vi "Test Get Report Path.vi"(8 "error in (no error)":errorcluster, 11 "Configuration Manager Test in":refnum<class "Configuration Manager Test.lvclass">) -> (0 "error out":errorcluster, 3 "Configuration Manager Test out":refnum<class "Configuration Manager Test.lvclass">)   [LabVIEW 2020, in "Configuration Manager Test.lvclass"]
uses:
  Configuration Manager Test.lvclass
  C:/Program Files (x86)/National Instruments/LabVIEW 2020/vi.lib/Astemes/LUnit/Core/LUnit Test Case/Test Case.lvclass
  <vilib>/Astemes/LUnit/Core/LUnit Test Case/Test Case.lvclass/Test Case.ctl
  da4b3e93-04f0-485b-8eef-eaf6a6b0a3f6.vi
  <vilib>/Astemes/LUnit/Core/LUnit Test Case/Private/Append Pass Result.vi
  <vilib>/Astemes/LUnit/Core/LUnit Test Case/Private/Append Fail Result.vi
  da4b3e93-04f0-485b-8eef-eaf6a6b0a3f6.vi/9c5d11cd-9439-4240-a1ee-d9baace9c924.vi
  <vilib>/Astemes/LUnit/Core/LUnit Test Case/Private/Run In UI.vi
  <vilib>/Utility/error.llb/Clear Errors.vi
  source/User Interface/Configuration Manager/Configuration Manager.lvclass
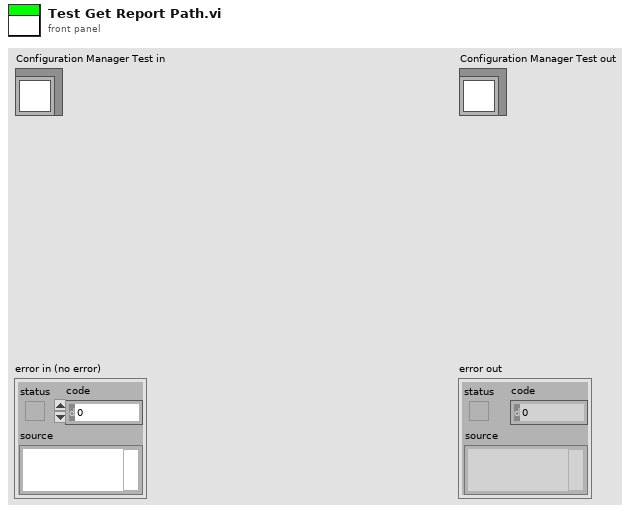
[diagram p1: front panel]
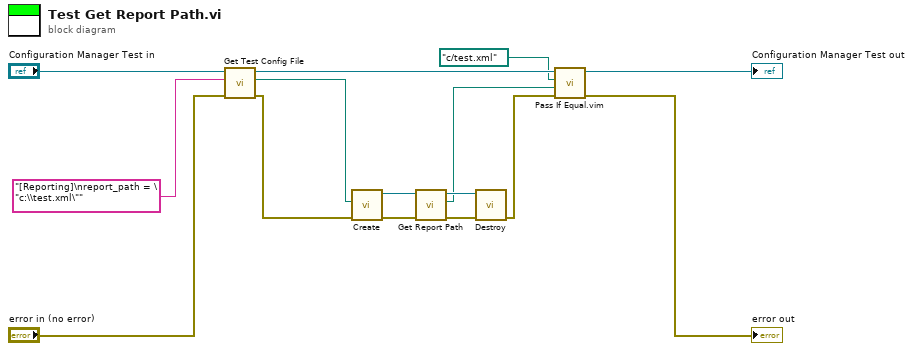
[diagram p0: block diagram]
diagram:
  n1 = call "Get Test Config File.vi"("error in (no error)"="error in (no error)", "File Content"="[Reporting]\nreport_path = \"c:\\test.xml\"", "Configuration Manager Test in"="Configuration Manager Test in") -> ("error out"=w8:errorcluster, "File Path"=w3:path, "Configuration Manager Test out"=w5:refnum<class "Configuration Manager Test.lvclass">)  [unwired: 6 in]
  n2 = call "Create.vi"("error in (no error)"=w8, "configuration file path"=w3) -> ("error out"=w11:errorcluster, "Configuration Manager out"=w12:refnum<class "Configuration Manager.lvclass">)  [unwired: 8 in]
  n3 = call "Get Report Path.vi"("error in (no error)"=w11, "Configuration Manager in"=w12) -> ("error out"=w9:errorcluster, "Report Path"=w1:path, "Configuration Manager out"=w10:refnum<class "Configuration Manager.lvclass">)  [unwired: 7 in]
  n4 = call "Destroy.vi"("error in (no error)"=w9, "Configuration Manager In"=w10) -> ("error out"=w7:errorcluster)  [unwired: 9 in]
  n5 = call "Pass If Equal.vim"("error in (no error)"=w7, "Actual"=w1, "Expected"=path "c:/test.xml" ("Report Path"), "LUnit Test Case In"=w5) -> ("error out"=→"error out":errorcluster, "LUnit Test Case Out"=→"Configuration Manager Test out":refnum<class "Configuration Manager Test.lvclass">)  [unwired: 6 in]
